vi "PatchCore_DS_Reader.vi"(4 "Read Bads?":bool, 5 "Input3D_Custom_Dims":T1, 6 "PreProcessing_Options":T2={"Image Type"=4, "Normalization Type"=enum."Standardize(DS_Stats)", "Interpolation Type"=1} {"Interpolation Type" items=["Zero Order", "Bi-Linear", "Quadratic", "Cubic Spline"]; "Image Type" items=["Grayscale (U8)", "Grayscale (I16)", "Grayscale (SGL)", "Complex (CSG)", "RGB (U32)", "HSL (U32)", "RGB (U64)", "Grayscale (U16)"]}, 7 "Dataset_Stats":T8={"means"={"R"=0.30100304, "G"=0.3015279, "B"=0.32350188}, "vars"={"R"=0.30371806, "G"=0.30376178, "B"=0.2861995}, "DS_Size"=0} {"vars"."R" format="%#_3g"; "vars"."G" format="%#_3g"; "vars"."B" format="%#_3g"; "means"."R" format="%#_3g"; "means"."G" format="%#_3g"; "means"."B" format="%#_3g"}, 8 "error in":errorcluster, 9 "GT Mask Folder Path":path, 10 "Bad Image File Paths":path[](array[path])=[path "D:/DNN/MVTec/pill/train/good/000.png", path "D:/DNN/MVTec/pill/train/good/001.png", path "D:/DNN/MVTec/pill/train/good/002.png", path "D:/DNN/MVTec/pill/train/good/003.png", path "D:/DNN/MVTec/pill/train/good/004.png", path "D:/DNN/MVTec/pill/train/good/005.png", path "D:/DNN/MVTec/pill/train/good/006.png", path "D:/DNN/MVTec/pill/train/good/007.png", path "D:/DNN/MVTec/pill/train/good/008.png", path "D:/DNN/MVTec/pill/train/good/009.png", path "D:/DNN/MVTec/pill/train/good/010.png", path "D:/DNN/MVTec/pill/train/good/011.png", path "D:/DNN/MVTec/pill/train/good/012.png", path "D:/DNN/MVTec/pill/train/good/013.png", path "D:/DNN/MVTec/pill/train/good/014.png", path "D:/DNN/MVTec/pill/train/good/015.png", path "D:/DNN/MVTec/pill/train/good/016.png", path "D:/DNN/MVTec/pill/train/good/017.png", path "D:/DNN/MVTec/pill/train/good/018.png", path "D:/DNN/MVTec/pill/train/good/019.png", path "D:/DNN/MVTec/pill/train/good/020.png", path "D:/DNN/MVTec/pill/train/good/021.png", path "D:/DNN/MVTec/pill/train/good/022.png", path "D:/DNN/MVTec/pill/train/good/023.png", path "D:/DNN/MVTec/pill/train/good/024.png", path "D:/DNN/MVTec/pill/train/good/025.png", path "D:/DNN/MVTec/pill/train/good/026.png", path "D:/DNN/MVTec/pill/train/good/027.png", path "D:/DNN/MVTec/pill/train/good/028.png", path "D:/DNN/MVTec/pill/train/good/029.png", path "D:/DNN/MVTec/pill/train/good/030.png", path "D:/DNN/MVTec/pill/train/good/031.png", path "D:/DNN/MVTec/pill/train/good/032.png", path "D:/DNN/MVTec/pill/train/good/033.png", path "D:/DNN/MVTec/pill/train/good/034.png", path "D:/DNN/MVTec/pill/train/good/035.png", path "D:/DNN/MVTec/pill/train/good/036.png", path "D:/DNN/MVTec/pill/train/good/037.png", path "D:/DNN/MVTec/pill/train/good/038.png", path "D:/DNN/MVTec/pill/train/good/039.png", path "D:/DNN/MVTec/pill/train/good/040.png", path "D:/DNN/MVTec/pill/train/good/041.png", path "D:/DNN/MVTec/pill/train/good/042.png", path "D:/DNN/MVTec/pill/train/good/043.png", path "D:/DNN/MVTec/pill/train/good/044.png", path "D:/DNN/MVTec/pill/train/good/045.png", path "D:/DNN/MVTec/pill/train/good/046.png", path "D:/DNN/MVTec/pill/train/good/047.png", path "D:/DNN/MVTec/pill/train/good/048.png", path "D:/DNN/MVTec/pill/train/good/049.png", path "D:/DNN/MVTec/pill/train/good/050.png", path "D:/DNN/MVTec/pill/train/good/051.png", path "D:/DNN/MVTec/pill/train/good/052.png", path "D:/DNN/MVTec/pill/train/good/053.png", path "D:/DNN/MVTec/pill/train/good/054.png", path "D:/DNN/MVTec/pill/train/good/055.png", path "D:/DNN/MVTec/pill/train/good/056.png", path "D:/DNN/MVTec/pill/train/good/057.png", path "D:/DNN/MVTec/pill/train/good/058.png", path "D:/DNN/MVTec/pill/train/good/059.png", path "D:/DNN/MVTec/pill/train/good/060.png", path "D:/DNN/MVTec/pill/train/good/061.png", path "D:/DNN/MVTec/pill/train/good/062.png", path "D:/DNN/MVTec/pill/train/good/063.png", path "D:/DNN/MVTec/pill/train/good/064.png", path "D:/DNN/MVTec/pill/train/good/065.png", path "D:/DNN/MVTec/pill/train/good/066.png", path "D:/DNN/MVTec/pill/train/good/067.png", path "D:/DNN/MVTec/pill/train/good/068.png", path "D:/DNN/MVTec/pill/train/good/069.png", path "D:/DNN/MVTec/pill/train/good/070.png", path "D:/DNN/MVTec/pill/train/good/071.png", path "D:/DNN/MVTec/pill/train/good/072.png", path "D:/DNN/MVTec/pill/train/good/073.png", path "D:/DNN/MVTec/pill/train/good/074.png", path "D:/DNN/MVTec/pill/train/good/075.png", path "D:/DNN/MVTec/pill/train/good/076.png", path "D:/DNN/MVTec/pill/train/good/077.png", path "D:/DNN/MVTec/pill/train/good/078.png", path "D:/DNN/MVTec/pill/train/good/079.png", path "D:/DNN/MVTec/pill/train/good/080.png", path "D:/DNN/MVTec/pill/train/good/081.png", path "D:/DNN/MVTec/pill/train/good/082.png", path "D:/DNN/MVTec/pill/train/good/083.png", path "D:/DNN/MVTec/pill/train/good/084.png", path "D:/DNN/MVTec/pill/train/good/085.png", path "D:/DNN/MVTec/pill/train/good/086.png", path "D:/DNN/MVTec/pill/train/good/087.png", path "D:/DNN/MVTec/pill/train/good/088.png", path "D:/DNN/MVTec/pill/train/good/089.png", path "D:/DNN/MVTec/pill/train/good/090.png", path "D:/DNN/MVTec/pill/train/good/091.png", path "D:/DNN/MVTec/pill/train/good/092.png", path "D:/DNN/MVTec/pill/train/good/093.png", path "D:/DNN/MVTec/pill/train/good/094.png", path "D:/DNN/MVTec/pill/train/good/095.png", path "D:/DNN/MVTec/pill/train/good/096.png", path "D:/DNN/MVTec/pill/train/good/097.png", path "D:/DNN/MVTec/pill/train/good/098.png", path "D:/DNN/MVTec/pill/train/good/099.png", path "D:/DNN/MVTec/pill/train/good/100.png", path "D:/DNN/MVTec/pill/train/good/101.png", path "D:/DNN/MVTec/pill/train/good/102.png", path "D:/DNN/MVTec/pill/train/good/103.png", path "D:/DNN/MVTec/pill/train/good/104.png", path "D:/DNN/MVTec/pill/train/good/105.png", path "D:/DNN/MVTec/pill/train/good/106.png", path "D:/DNN/MVTec/pill/train/good/107.png", path "D:/DNN/MVTec/pill/train/good/108.png", path "D:/DNN/MVTec/pill/train/good/109.png", path "D:/DNN/MVTec/pill/train/good/110.png", path "D:/DNN/MVTec/pill/train/good/111.png", path "D:/DNN/MVTec/pill/train/good/112.png", path "D:/DNN/MVTec/pill/train/good/113.png", path "D:/DNN/MVTec/pill/train/good/114.png", path "D:/DNN/MVTec/pill/train/good/115.png", path "D:/DNN/MVTec/pill/train/good/116.png", path "D:/DNN/MVTec/pill/train/good/117.png", path "D:/DNN/MVTec/pill/train/good/118.png", path "D:/DNN/MVTec/pill/train/good/119.png", path "D:/DNN/MVTec/pill/train/good/120.png", path "D:/DNN/MVTec/pill/train/good/121.png", path "D:/DNN/MVTec/pill/train/good/122.png", path "D:/DNN/MVTec/pill/train/good/123.png", path "D:/DNN/MVTec/pill/train/good/124.png", path "D:/DNN/MVTec/pill/train/good/125.png", path "D:/DNN/MVTec/pill/train/good/126.png", path "D:/DNN/MVTec/pill/train/good/127.png", path "D:/DNN/MVTec/pill/train/good/128.png", path "D:/DNN/MVTec/pill/train/good/129.png", path "D:/DNN/MVTec/pill/train/good/130.png", path "D:/DNN/MVTec/pill/train/good/131.png", path "D:/DNN/MVTec/pill/train/good/132.png", path "D:/DNN/MVTec/pill/train/good/133.png", path "D:/DNN/MVTec/pill/train/good/134.png", path "D:/DNN/MVTec/pill/train/good/135.png", path "D:/DNN/MVTec/pill/train/good/136.png", path "D:/DNN/MVTec/pill/train/good/137.png", path "D:/DNN/MVTec/pill/train/good/138.png", path "D:/DNN/MVTec/pill/train/good/139.png", path "D:/DNN/MVTec/pill/train/good/140.png", path "D:/DNN/MVTec/pill/train/good/141.png", path "D:/DNN/MVTec/pill/train/good/142.png", path "D:/DNN/MVTec/pill/train/good/143.png", path "D:/DNN/MVTec/pill/train/good/144.png", path "D:/DNN/MVTec/pill/train/good/145.png", path "D:/DNN/MVTec/pill/train/good/146.png", path "D:/DNN/MVTec/pill/train/good/147.png", path "D:/DNN/MVTec/pill/train/good/148.png", path "D:/DNN/MVTec/pill/train/good/149.png", path "D:/DNN/MVTec/pill/train/good/150.png", path "D:/DNN/MVTec/pill/train/good/151.png", path "D:/DNN/MVTec/pill/train/good/152.png", path "D:/DNN/MVTec/pill/train/good/153.png", path "D:/DNN/MVTec/pill/train/good/154.png", path "D:/DNN/MVTec/pill/train/good/155.png", path "D:/DNN/MVTec/pill/train/good/156.png", path "D:/DNN/MVTec/pill/train/good/157.png", path "D:/DNN/MVTec/pill/train/good/158.png", path "D:/DNN/MVTec/pill/train/good/159.png", path "D:/DNN/MVTec/pill/train/good/160.png", path "D:/DNN/MVTec/pill/train/good/161.png", path "D:/DNN/MVTec/pill/train/good/162.png", path "D:/DNN/MVTec/pill/train/good/163.png", path "D:/DNN/MVTec/pill/train/good/164.png", path "D:/DNN/MVTec/pill/train/good/165.png", path "D:/DNN/MVTec/pill/train/good/166.png", path "D:/DNN/MVTec/pill/train/good/167.png", path "D:/DNN/MVTec/pill/train/good/168.png", path "D:/DNN/MVTec/pill/train/good/169.png", path "D:/DNN/MVTec/pill/train/good/170.png", path "D:/DNN/MVTec/pill/train/good/171.png", path "D:/DNN/MVTec/pill/train/good/172.png", path "D:/DNN/MVTec/pill/train/good/173.png", path "D:/DNN/MVTec/pill/train/good/174.png", path "D:/DNN/MVTec/pill/train/good/175.png", path "D:/DNN/MVTec/pill/train/good/176.png", path "D:/DNN/MVTec/pill/train/good/177.png", path "D:/DNN/MVTec/pill/train/good/178.png", path "D:/DNN/MVTec/pill/train/good/179.png", path "D:/DNN/MVTec/pill/train/good/180.png", path "D:/DNN/MVTec/pill/train/good/181.png", path "D:/DNN/MVTec/pill/train/good/182.png", path "D:/DNN/MVTec/pill/train/good/183.png", path "D:/DNN/MVTec/pill/train/good/184.png", path "D:/DNN/MVTec/pill/train/good/185.png", path "D:/DNN/MVTec/pill/train/good/186.png", path "D:/DNN/MVTec/pill/train/good/187.png", path "D:/DNN/MVTec/pill/train/good/188.png", path "D:/DNN/MVTec/pill/train/good/189.png", path "D:/DNN/MVTec/pill/train/good/190.png", path "D:/DNN/MVTec/pill/train/good/191.png", path "D:/DNN/MVTec/pill/train/good/192.png", path "D:/DNN/MVTec/pill/train/good/193.png", path "D:/DNN/MVTec/pill/train/good/194.png", path "D:/DNN/MVTec/pill/train/good/195.png", path "D:/DNN/MVTec/pill/train/good/196.png", path "D:/DNN/MVTec/pill/train/good/197.png", path "D:/DNN/MVTec/pill/train/good/198.png", path "D:/DNN/MVTec/pill/train/good/199.png", path "D:/DNN/MVTec/pill/train/good/200.png", path "D:/DNN/MVTec/pill/train/good/201.png", path "D:/DNN/MVTec/pill/train/good/202.png", path "D:/DNN/MVTec/pill/train/good/203.png", path "D:/DNN/MVTec/pill/train/good/204.png", path "D:/DNN/MVTec/pill/train/good/205.png", path "D:/DNN/MVTec/pill/train/good/206.png", path "D:/DNN/MVTec/pill/train/good/207.png", path "D:/DNN/MVTec/pill/train/good/208.png", path "D:/DNN/MVTec/pill/train/good/209.png", path "D:/DNN/MVTec/pill/train/good/210.png", path "D:/DNN/MVTec/pill/train/good/211.png", path "D:/DNN/MVTec/pill/train/good/212.png", path "D:/DNN/MVTec/pill/train/good/213.png", path "D:/DNN/MVTec/pill/train/good/214.png", path "D:/DNN/MVTec/pill/train/good/215.png", path "D:/DNN/MVTec/pill/train/good/216.png", path "D:/DNN/MVTec/pill/train/good/217.png", path "D:/DNN/MVTec/pill/train/good/218.png", path "D:/DNN/MVTec/pill/train/good/219.png", path "D:/DNN/MVTec/pill/train/good/220.png", path "D:/DNN/MVTec/pill/train/good/221.png", path "D:/DNN/MVTec/pill/train/good/222.png", path "D:/DNN/MVTec/pill/train/good/223.png", path "D:/DNN/MVTec/pill/train/good/224.png", path "D:/DNN/MVTec/pill/train/good/225.png", path "D:/DNN/MVTec/pill/train/good/226.png", path "D:/DNN/MVTec/pill/train/good/227.png", path "D:/DNN/MVTec/pill/train/good/228.png", path "D:/DNN/MVTec/pill/train/good/229.png", path "D:/DNN/MVTec/pill/train/good/230.png", path "D:/DNN/MVTec/pill/train/good/231.png", path "D:/DNN/MVTec/pill/train/good/232.png", path "D:/DNN/MVTec/pill/train/good/233.png", path "D:/DNN/MVTec/pill/train/good/234.png", path "D:/DNN/MVTec/pill/train/good/235.png", path "D:/DNN/MVTec/pill/train/good/236.png", path "D:/DNN/MVTec/pill/train/good/237.png", path "D:/DNN/MVTec/pill/train/good/238.png", path "D:/DNN/MVTec/pill/train/good/239.png", path "D:/DNN/MVTec/pill/train/good/240.png", path "D:/DNN/MVTec/pill/train/good/241.png", path "D:/DNN/MVTec/pill/train/good/242.png", path "D:/DNN/MVTec/pill/train/good/243.png", path "D:/DNN/MVTec/pill/train/good/244.png", path "D:/DNN/MVTec/pill/train/good/245.png", path "D:/DNN/MVTec/pill/train/good/246.png", path "D:/DNN/MVTec/pill/train/good/247.png", path "D:/DNN/MVTec/pill/train/good/248.png", path "D:/DNN/MVTec/pill/train/good/249.png", path "D:/DNN/MVTec/pill/train/good/250.png", path "D:/DNN/MVTec/pill/train/good/251.png", path "D:/DNN/MVTec/pill/train/good/252.png", path "D:/DNN/MVTec/pill/train/good/253.png", path "D:/DNN/MVTec/pill/train/good/254.png", path "D:/DNN/MVTec/pill/train/good/255.png", path "D:/DNN/MVTec/pill/train/good/256.png", path "D:/DNN/MVTec/pill/train/good/257.png", path "D:/DNN/MVTec/pill/train/good/258.png", path "D:/DNN/MVTec/pill/train/good/259.png", path "D:/DNN/MVTec/pill/train/good/260.png", path "D:/DNN/MVTec/pill/train/good/261.png", path "D:/DNN/MVTec/pill/train/good/262.png", path "D:/DNN/MVTec/pill/train/good/263.png", path "D:/DNN/MVTec/pill/train/good/264.png", path "D:/DNN/MVTec/pill/train/good/265.png", path "D:/DNN/MVTec/pill/train/good/266.png"], 11 "Good Image File Paths":path[](array[path])=[path "D:/DNN/MVTec/pill/train/good/000.png", path "D:/DNN/MVTec/pill/train/good/001.png", path "D:/DNN/MVTec/pill/train/good/002.png", path "D:/DNN/MVTec/pill/train/good/003.png", path "D:/DNN/MVTec/pill/train/good/004.png", path "D:/DNN/MVTec/pill/train/good/005.png", path "D:/DNN/MVTec/pill/train/good/006.png", path "D:/DNN/MVTec/pill/train/good/007.png", path "D:/DNN/MVTec/pill/train/good/008.png", path "D:/DNN/MVTec/pill/train/good/009.png", path "D:/DNN/MVTec/pill/train/good/010.png", path "D:/DNN/MVTec/pill/train/good/011.png", path "D:/DNN/MVTec/pill/train/good/012.png", path "D:/DNN/MVTec/pill/train/good/013.png", path "D:/DNN/MVTec/pill/train/good/014.png", path "D:/DNN/MVTec/pill/train/good/015.png", path "D:/DNN/MVTec/pill/train/good/016.png", path "D:/DNN/MVTec/pill/train/good/017.png", path "D:/DNN/MVTec/pill/train/good/018.png", path "D:/DNN/MVTec/pill/train/good/019.png", path "D:/DNN/MVTec/pill/train/good/020.png", path "D:/DNN/MVTec/pill/train/good/021.png", path "D:/DNN/MVTec/pill/train/good/022.png", path "D:/DNN/MVTec/pill/train/good/023.png", path "D:/DNN/MVTec/pill/train/good/024.png", path "D:/DNN/MVTec/pill/train/good/025.png", path "D:/DNN/MVTec/pill/train/good/026.png", path "D:/DNN/MVTec/pill/train/good/027.png", path "D:/DNN/MVTec/pill/train/good/028.png", path "D:/DNN/MVTec/pill/train/good/029.png", path "D:/DNN/MVTec/pill/train/good/030.png", path "D:/DNN/MVTec/pill/train/good/031.png", path "D:/DNN/MVTec/pill/train/good/032.png", path "D:/DNN/MVTec/pill/train/good/033.png", path "D:/DNN/MVTec/pill/train/good/034.png", path "D:/DNN/MVTec/pill/train/good/035.png", path "D:/DNN/MVTec/pill/train/good/036.png", path "D:/DNN/MVTec/pill/train/good/037.png", path "D:/DNN/MVTec/pill/train/good/038.png", path "D:/DNN/MVTec/pill/train/good/039.png", path "D:/DNN/MVTec/pill/train/good/040.png", path "D:/DNN/MVTec/pill/train/good/041.png", path "D:/DNN/MVTec/pill/train/good/042.png", path "D:/DNN/MVTec/pill/train/good/043.png", path "D:/DNN/MVTec/pill/train/good/044.png", path "D:/DNN/MVTec/pill/train/good/045.png", path "D:/DNN/MVTec/pill/train/good/046.png", path "D:/DNN/MVTec/pill/train/good/047.png", path "D:/DNN/MVTec/pill/train/good/048.png", path "D:/DNN/MVTec/pill/train/good/049.png", path "D:/DNN/MVTec/pill/train/good/050.png", path "D:/DNN/MVTec/pill/train/good/051.png", path "D:/DNN/MVTec/pill/train/good/052.png", path "D:/DNN/MVTec/pill/train/good/053.png", path "D:/DNN/MVTec/pill/train/good/054.png", path "D:/DNN/MVTec/pill/train/good/055.png", path "D:/DNN/MVTec/pill/train/good/056.png", path "D:/DNN/MVTec/pill/train/good/057.png", path "D:/DNN/MVTec/pill/train/good/058.png", path "D:/DNN/MVTec/pill/train/good/059.png", path "D:/DNN/MVTec/pill/train/good/060.png", path "D:/DNN/MVTec/pill/train/good/061.png", path "D:/DNN/MVTec/pill/train/good/062.png", path "D:/DNN/MVTec/pill/train/good/063.png", path "D:/DNN/MVTec/pill/train/good/064.png", path "D:/DNN/MVTec/pill/train/good/065.png", path "D:/DNN/MVTec/pill/train/good/066.png", path "D:/DNN/MVTec/pill/train/good/067.png", path "D:/DNN/MVTec/pill/train/good/068.png", path "D:/DNN/MVTec/pill/train/good/069.png", path "D:/DNN/MVTec/pill/train/good/070.png", path "D:/DNN/MVTec/pill/train/good/071.png", path "D:/DNN/MVTec/pill/train/good/072.png", path "D:/DNN/MVTec/pill/train/good/073.png", path "D:/DNN/MVTec/pill/train/good/074.png", path "D:/DNN/MVTec/pill/train/good/075.png", path "D:/DNN/MVTec/pill/train/good/076.png", path "D:/DNN/MVTec/pill/train/good/077.png", path "D:/DNN/MVTec/pill/train/good/078.png", path "D:/DNN/MVTec/pill/train/good/079.png", path "D:/DNN/MVTec/pill/train/good/080.png", path "D:/DNN/MVTec/pill/train/good/081.png", path "D:/DNN/MVTec/pill/train/good/082.png", path "D:/DNN/MVTec/pill/train/good/083.png", path "D:/DNN/MVTec/pill/train/good/084.png", path "D:/DNN/MVTec/pill/train/good/085.png", path "D:/DNN/MVTec/pill/train/good/086.png", path "D:/DNN/MVTec/pill/train/good/087.png", path "D:/DNN/MVTec/pill/train/good/088.png", path "D:/DNN/MVTec/pill/train/good/089.png", path "D:/DNN/MVTec/pill/train/good/090.png", path "D:/DNN/MVTec/pill/train/good/091.png", path "D:/DNN/MVTec/pill/train/good/092.png", path "D:/DNN/MVTec/pill/train/good/093.png", path "D:/DNN/MVTec/pill/train/good/094.png", path "D:/DNN/MVTec/pill/train/good/095.png", path "D:/DNN/MVTec/pill/train/good/096.png", path "D:/DNN/MVTec/pill/train/good/097.png", path "D:/DNN/MVTec/pill/train/good/098.png", path "D:/DNN/MVTec/pill/train/good/099.png", path "D:/DNN/MVTec/pill/train/good/100.png", path "D:/DNN/MVTec/pill/train/good/101.png", path "D:/DNN/MVTec/pill/train/good/102.png", path "D:/DNN/MVTec/pill/train/good/103.png", path "D:/DNN/MVTec/pill/train/good/104.png", path "D:/DNN/MVTec/pill/train/good/105.png", path "D:/DNN/MVTec/pill/train/good/106.png", path "D:/DNN/MVTec/pill/train/good/107.png", path "D:/DNN/MVTec/pill/train/good/108.png", path "D:/DNN/MVTec/pill/train/good/109.png", path "D:/DNN/MVTec/pill/train/good/110.png", path "D:/DNN/MVTec/pill/train/good/111.png", path "D:/DNN/MVTec/pill/train/good/112.png", path "D:/DNN/MVTec/pill/train/good/113.png", path "D:/DNN/MVTec/pill/train/good/114.png", path "D:/DNN/MVTec/pill/train/good/115.png", path "D:/DNN/MVTec/pill/train/good/116.png", path "D:/DNN/MVTec/pill/train/good/117.png", path "D:/DNN/MVTec/pill/train/good/118.png", path "D:/DNN/MVTec/pill/train/good/119.png", path "D:/DNN/MVTec/pill/train/good/120.png", path "D:/DNN/MVTec/pill/train/good/121.png", path "D:/DNN/MVTec/pill/train/good/122.png", path "D:/DNN/MVTec/pill/train/good/123.png", path "D:/DNN/MVTec/pill/train/good/124.png", path "D:/DNN/MVTec/pill/train/good/125.png", path "D:/DNN/MVTec/pill/train/good/126.png", path "D:/DNN/MVTec/pill/train/good/127.png", path "D:/DNN/MVTec/pill/train/good/128.png", path "D:/DNN/MVTec/pill/train/good/129.png", path "D:/DNN/MVTec/pill/train/good/130.png", path "D:/DNN/MVTec/pill/train/good/131.png", path "D:/DNN/MVTec/pill/train/good/132.png", path "D:/DNN/MVTec/pill/train/good/133.png", path "D:/DNN/MVTec/pill/train/good/134.png", path "D:/DNN/MVTec/pill/train/good/135.png", path "D:/DNN/MVTec/pill/train/good/136.png", path "D:/DNN/MVTec/pill/train/good/137.png", path "D:/DNN/MVTec/pill/train/good/138.png", path "D:/DNN/MVTec/pill/train/good/139.png", path "D:/DNN/MVTec/pill/train/good/140.png", path "D:/DNN/MVTec/pill/train/good/141.png", path "D:/DNN/MVTec/pill/train/good/142.png", path "D:/DNN/MVTec/pill/train/good/143.png", path "D:/DNN/MVTec/pill/train/good/144.png", path "D:/DNN/MVTec/pill/train/good/145.png", path "D:/DNN/MVTec/pill/train/good/146.png", path "D:/DNN/MVTec/pill/train/good/147.png", path "D:/DNN/MVTec/pill/train/good/148.png", path "D:/DNN/MVTec/pill/train/good/149.png", path "D:/DNN/MVTec/pill/train/good/150.png", path "D:/DNN/MVTec/pill/train/good/151.png", path "D:/DNN/MVTec/pill/train/good/152.png", path "D:/DNN/MVTec/pill/train/good/153.png", path "D:/DNN/MVTec/pill/train/good/154.png", path "D:/DNN/MVTec/pill/train/good/155.png", path "D:/DNN/MVTec/pill/train/good/156.png", path "D:/DNN/MVTec/pill/train/good/157.png", path "D:/DNN/MVTec/pill/train/good/158.png", path "D:/DNN/MVTec/pill/train/good/159.png", path "D:/DNN/MVTec/pill/train/good/160.png", path "D:/DNN/MVTec/pill/train/good/161.png", path "D:/DNN/MVTec/pill/train/good/162.png", path "D:/DNN/MVTec/pill/train/good/163.png", path "D:/DNN/MVTec/pill/train/good/164.png", path "D:/DNN/MVTec/pill/train/good/165.png", path "D:/DNN/MVTec/pill/train/good/166.png", path "D:/DNN/MVTec/pill/train/good/167.png", path "D:/DNN/MVTec/pill/train/good/168.png", path "D:/DNN/MVTec/pill/train/good/169.png", path "D:/DNN/MVTec/pill/train/good/170.png", path "D:/DNN/MVTec/pill/train/good/171.png", path "D:/DNN/MVTec/pill/train/good/172.png", path "D:/DNN/MVTec/pill/train/good/173.png", path "D:/DNN/MVTec/pill/train/good/174.png", path "D:/DNN/MVTec/pill/train/good/175.png", path "D:/DNN/MVTec/pill/train/good/176.png", path "D:/DNN/MVTec/pill/train/good/177.png", path "D:/DNN/MVTec/pill/train/good/178.png", path "D:/DNN/MVTec/pill/train/good/179.png", path "D:/DNN/MVTec/pill/train/good/180.png", path "D:/DNN/MVTec/pill/train/good/181.png", path "D:/DNN/MVTec/pill/train/good/182.png", path "D:/DNN/MVTec/pill/train/good/183.png", path "D:/DNN/MVTec/pill/train/good/184.png", path "D:/DNN/MVTec/pill/train/good/185.png", path "D:/DNN/MVTec/pill/train/good/186.png", path "D:/DNN/MVTec/pill/train/good/187.png", path "D:/DNN/MVTec/pill/train/good/188.png", path "D:/DNN/MVTec/pill/train/good/189.png", path "D:/DNN/MVTec/pill/train/good/190.png", path "D:/DNN/MVTec/pill/train/good/191.png", path "D:/DNN/MVTec/pill/train/good/192.png", path "D:/DNN/MVTec/pill/train/good/193.png", path "D:/DNN/MVTec/pill/train/good/194.png", path "D:/DNN/MVTec/pill/train/good/195.png", path "D:/DNN/MVTec/pill/train/good/196.png", path "D:/DNN/MVTec/pill/train/good/197.png", path "D:/DNN/MVTec/pill/train/good/198.png", path "D:/DNN/MVTec/pill/train/good/199.png", path "D:/DNN/MVTec/pill/train/good/200.png", path "D:/DNN/MVTec/pill/train/good/201.png", path "D:/DNN/MVTec/pill/train/good/202.png", path "D:/DNN/MVTec/pill/train/good/203.png", path "D:/DNN/MVTec/pill/train/good/204.png", path "D:/DNN/MVTec/pill/train/good/205.png", path "D:/DNN/MVTec/pill/train/good/206.png", path "D:/DNN/MVTec/pill/train/good/207.png", path "D:/DNN/MVTec/pill/train/good/208.png", path "D:/DNN/MVTec/pill/train/good/209.png", path "D:/DNN/MVTec/pill/train/good/210.png", path "D:/DNN/MVTec/pill/train/good/211.png", path "D:/DNN/MVTec/pill/train/good/212.png", path "D:/DNN/MVTec/pill/train/good/213.png", path "D:/DNN/MVTec/pill/train/good/214.png", path "D:/DNN/MVTec/pill/train/good/215.png", path "D:/DNN/MVTec/pill/train/good/216.png", path "D:/DNN/MVTec/pill/train/good/217.png", path "D:/DNN/MVTec/pill/train/good/218.png", path "D:/DNN/MVTec/pill/train/good/219.png", path "D:/DNN/MVTec/pill/train/good/220.png", path "D:/DNN/MVTec/pill/train/good/221.png", path "D:/DNN/MVTec/pill/train/good/222.png", path "D:/DNN/MVTec/pill/train/good/223.png", path "D:/DNN/MVTec/pill/train/good/224.png", path "D:/DNN/MVTec/pill/train/good/225.png", path "D:/DNN/MVTec/pill/train/good/226.png", path "D:/DNN/MVTec/pill/train/good/227.png", path "D:/DNN/MVTec/pill/train/good/228.png", path "D:/DNN/MVTec/pill/train/good/229.png", path "D:/DNN/MVTec/pill/train/good/230.png", path "D:/DNN/MVTec/pill/train/good/231.png", path "D:/DNN/MVTec/pill/train/good/232.png", path "D:/DNN/MVTec/pill/train/good/233.png", path "D:/DNN/MVTec/pill/train/good/234.png", path "D:/DNN/MVTec/pill/train/good/235.png", path "D:/DNN/MVTec/pill/train/good/236.png", path "D:/DNN/MVTec/pill/train/good/237.png", path "D:/DNN/MVTec/pill/train/good/238.png", path "D:/DNN/MVTec/pill/train/good/239.png", path "D:/DNN/MVTec/pill/train/good/240.png", path "D:/DNN/MVTec/pill/train/good/241.png", path "D:/DNN/MVTec/pill/train/good/242.png", path "D:/DNN/MVTec/pill/train/good/243.png", path "D:/DNN/MVTec/pill/train/good/244.png", path "D:/DNN/MVTec/pill/train/good/245.png", path "D:/DNN/MVTec/pill/train/good/246.png", path "D:/DNN/MVTec/pill/train/good/247.png", path "D:/DNN/MVTec/pill/train/good/248.png", path "D:/DNN/MVTec/pill/train/good/249.png", path "D:/DNN/MVTec/pill/train/good/250.png", path "D:/DNN/MVTec/pill/train/good/251.png", path "D:/DNN/MVTec/pill/train/good/252.png", path "D:/DNN/MVTec/pill/train/good/253.png", path "D:/DNN/MVTec/pill/train/good/254.png", path "D:/DNN/MVTec/pill/train/good/255.png", path "D:/DNN/MVTec/pill/train/good/256.png", path "D:/DNN/MVTec/pill/train/good/257.png", path "D:/DNN/MVTec/pill/train/good/258.png", path "D:/DNN/MVTec/pill/train/good/259.png", path "D:/DNN/MVTec/pill/train/good/260.png", path "D:/DNN/MVTec/pill/train/good/261.png", path "D:/DNN/MVTec/pill/train/good/262.png", path "D:/DNN/MVTec/pill/train/good/263.png", path "D:/DNN/MVTec/pill/train/good/264.png", path "D:/DNN/MVTec/pill/train/good/265.png", path "D:/DNN/MVTec/pill/train/good/266.png"]) -> (0 "error out":errorcluster, 3 "Dataset":T5={"Train"={"Dataset_Size"=0, "Dims_In"={"C"=0, "H"=0, "W"=0}, "Labels"=[], "File Paths"=[], "Outputs Ref."=refnum, "Inputs Ref."=variant(refnum<data-value> refnum), "Dims_Out"={"C"=0, "H"=0, "W"=0}}, "Validation"={"Dataset_Size"=0, "Dims_In"={"C"=0, "H"=0, "W"=0}, "Labels"=[], "File Paths"=[], "Outputs Ref."=refnum, "Inputs Ref."=variant(refnum<data-value> refnum), "Dims_Out"={"C"=0, "H"=0, "W"=0}}, "Test"={"Dataset_Size"=0, "Dims_In"={"C"=0, "H"=0, "W"=0}, "Labels"=[], "File Paths"=[], "Outputs Ref."=refnum, "Inputs Ref."=variant(refnum<data-value> refnum), "Dims_Out"={"C"=0, "H"=0, "W"=0}}})   [LabVIEW 2020]
uses:
  PatchCore_AddOn/API/Controls/NNPC_DS_Stats.ctl
  PatchCore_AddOn/API/Controls/Image_Stats_RGB.ctl
  <vilib>/Ngene/Deep Learning Toolkit/Toolkit/NN_Data/API/DataSet/DataSet_Types/NN_DataSets_All(In3D_Out3D).ctl
  <vilib>/Ngene/Deep Learning Toolkit/Toolkit/NN_Data/API/DataSet/DataSet_Types/NN_DataSet(In3D_Out3D).ctl
  <vilib>/Ngene/Deep Learning Toolkit/Toolkit/NN_Data/API/NN_Dims(C,H,W).ctl
  <vilib>/Ngene/Deep Learning Toolkit/Toolkit/NN_Data/Controls/DataRef_Types/4D/NN_Data_ref(4D_SGL).ctl
  Controls/ImRead_PreProcessing_Options.ctl
  PatchCore_AddOn/Low_Level/Controls/Normalization_Type.ctl
  <vilib>/Ngene/Deep Learning Toolkit/Toolkit/Deep_Learning_Toolkit_by_Ngene.lvlib
  PatchCore_AddOn/PatchCore_AddOn.lvlib
panel:
  in  "Good Unique Labels":string[](array[string])
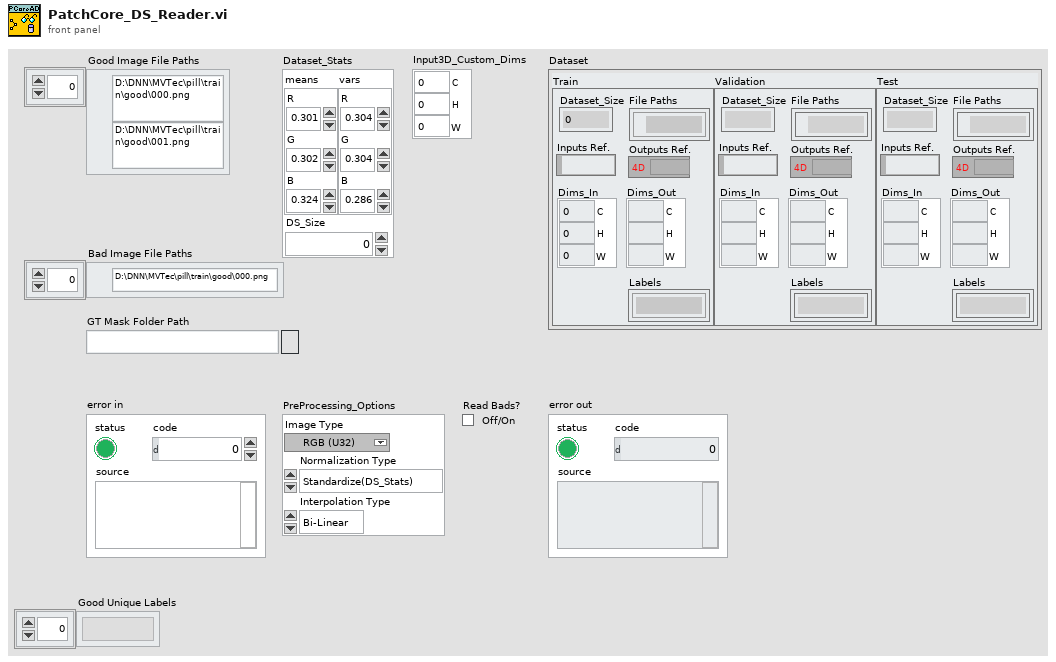
[diagram p1: front panel]
types:
  T1 = typedef "Deep_Learning_Toolkit_by_Ngene.lvlib/NN_Dims(C,H,W).ctl" = cluster{"C":i32, "H":i32, "W":i32}
  T2 = typedef "ImRead_PreProcessing_Options.ctl" = cluster{"Image Type":T3, "Normalization Type":T4, "Interpolation Type":u32}
  T3 = typedef "Image Type" = u32
  T4 = typedef "PatchCore_AddOn.lvlib/Normalization_Type.ctl" = enum16{"Standardize(DS_Stats)", "Standardize(Image_Stats)"}
  T5 = typedef "Deep_Learning_Toolkit_by_Ngene.lvlib/NN_DataSets_All(In3D_Out3D).ctl" = cluster{"Train":T6, "Validation":T6, "Test":T6}
  T6 = typedef "Deep_Learning_Toolkit_by_Ngene.lvlib/NN_DataSet(In3D_Out3D).ctl" = cluster{"Dataset_Size":i32, "Dims_In":T1, "Labels":string[], "File Paths":path[], "Outputs Ref.":T7, "Inputs Ref.":variant, "Dims_Out":T1}
  T7 = typedef "Deep_Learning_Toolkit_by_Ngene.lvlib/NN_Data_ref(4D_SGL).ctl" = refnum<data-value>
  T8 = typedef "PatchCore_AddOn.lvlib/NNPC_DS_Stats.ctl" = cluster{"means":T9, "vars":T9, "DS_Size":i32}
  T9 = typedef "PatchCore_AddOn.lvlib/Image_Stats_RGB.ctl" = cluster{"R":sgl, "G":sgl, "B":sgl}
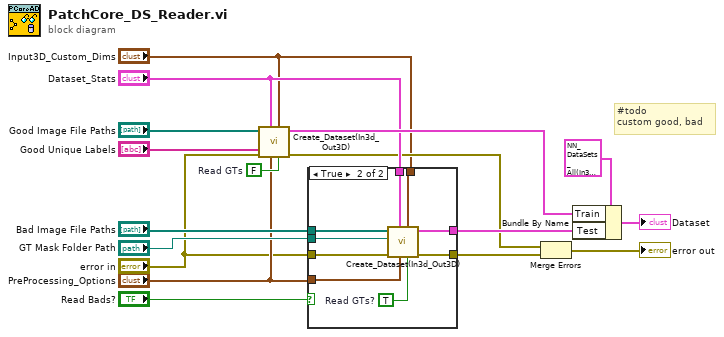
[diagram p0: block diagram]
diagram:
  w6 = FALSE  # Read GTs
  # "#todo\ncustom good, bad"
  n1 = call "Create_Dataset(In3d_Out3D).vi"("Read GTs?"=w6, "Input3D_Custom_Dims"="Input3D_Custom_Dims", "PreProcessing_Options"="PreProcessing_Options", "Dataset_Stats"="Dataset_Stats", "error in (no error)"="error in", "Good Unique Labels"="Good Unique Labels", "Image File Paths"="Good Image File Paths") -> ("error out"=w3:errorcluster, "Dataset(In3D_Out3D)"=w15:T6)  [unwired: 3 in]
  n2 = case shown="True" "Read Bads?" {
    tunnel: [w18 w27] -> w13
    tunnel: "GT Mask Folder Path" -> [_ w26]
    tunnel: "Bad Image File Paths" -> [_ w25]
    tunnel: "Dataset_Stats" -> [_ w24]
    tunnel: [_ w23] -> w7
    tunnel: "PreProcessing_Options" -> [_ w22]
    tunnel: "error in" -> [w18 w21]
    tunnel: "Input3D_Custom_Dims" -> [_ w19]
    frame False {
    }
    frame True {
      w20 = TRUE  # Read GTs?
      n3 = call "Create_Dataset(In3d_Out3D).vi"("Read GTs?"=w20, "Input3D_Custom_Dims"=w19, "PreProcessing_Options"=w22, "Dataset_Stats"=w24, "error in (no error)"=w21, "GT Folder Path"=w26, "Image File Paths"=w25) -> ("error out"=w27:errorcluster, "Dataset(In3D_Out3D)"=w23:T6)  [unwired: 3 in]
    }
  }
  n4 = Merge Errors(w3, w13) -> (→"error out":errorcluster)
  n5 = Bundle By Name(cluster=T5 {"Train"={"Dataset_Size"=0, "Dims_In"={"C"=0, "H"=0, "W"=0}, "Labels"=[], "File Paths"=[], "Outputs Ref."=refnum, "Inputs Ref."=variant(refnum<data-value> refnum), "Dims_Out"={"C"=0, "H"=0, "W"=0}}, "Validation"={"Dataset_Size"=0, "Dims_In"={"C"=0, "H"=0, "W"=0}, "Labels"=[], "File Paths"=[], "Outputs Ref."=refnum, "Inputs Ref."=variant(refnum<data-value> refnum), "Dims_Out"={"C"=0, "H"=0, "W"=0}}, "Test"={"Dataset_Size"=0, "Dims_In"={"C"=0, "H"=0, "W"=0}, "Labels"=[], "File Paths"=[], "Outputs Ref."=refnum, "Inputs Ref."=variant(refnum<data-value> refnum), "Dims_Out"={"C"=0, "H"=0, "W"=0}}} ("Datasets_All(In3D_Out3D)"), "Train"=w15, "Test"=w7) -> (→"Dataset":T5)
